vi "launch_auto2_test .vi"(7 "枚举":T1, 8 "error in (no error)":errorcluster, 9 "user event out":T2, 10 "modbusData":refnum<notifier>, 11 "Cluster":T3) -> (0 "error out":errorcluster)   [LabVIEW 2019]
uses:
  core_dataRefCluster.ctl
  core_dataRef.ctl
  core_dataCluster.ctl
  instrument/instr_dataCluster.ctl
  gui/test_result_user_event.ctl
  core_autoMonitorDataCluster.ctl
  gui/Enum.ctl
  instrument/Instrument.lvclass
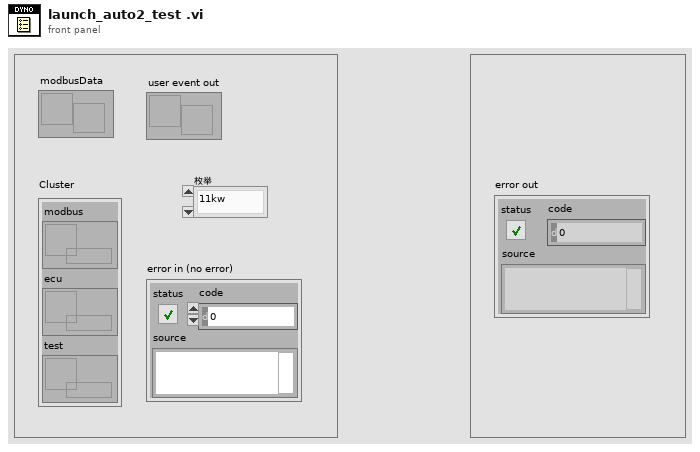
[diagram p1: front panel]
types:
  T1 = typedef "Enum.ctl" = enum16{"11kw", "5KW", "3.5KW"}
  T2 = typedef "test_result_user_event.ctl" = refnum<user-event>
  T3 = typedef "core_dataRefCluster.ctl" = cluster{"modbus":T4, "ecu":T4, "test":T4}
  T4 = typedef "core_dataRef.ctl" = refnum<queue>
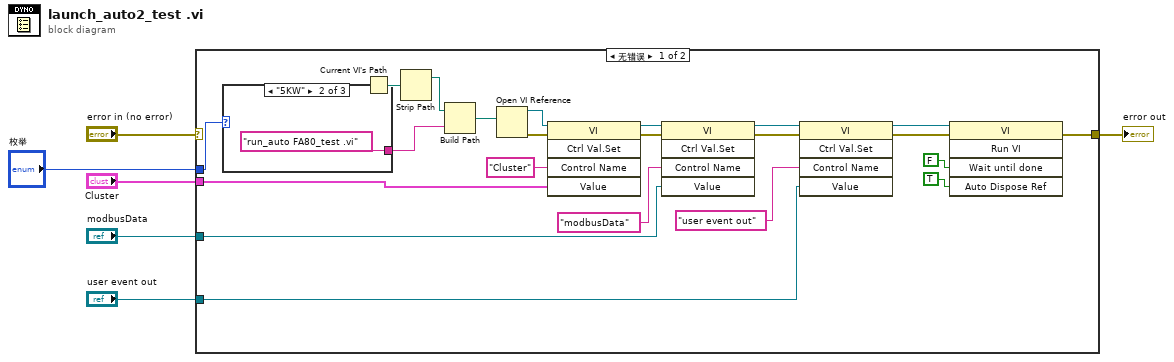
[diagram p0: block diagram]
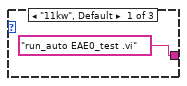
[diagram p2: hidden frame]
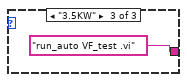
[diagram p3: hidden frame]
diagram:
  n1 = case shown="无错误" "error in (no error)" {
    selector: "error in (no error)" -> [_ w32]
    tunnel: "Cluster" -> [w26 _]
    tunnel: "modbusData" -> [w25 _]
    tunnel: [w15 w32] -> w4
    tunnel: "user event out" -> [w9 _]
    tunnel: "枚举" -> [w7 _]
    frame No Error {
      n2 = case shown="\"5KW\"" w7 {
        tunnel: ["run_auto EAE0_test .vi" ("name or relative path") "run_auto FA80_test .vi" ("name or relative path") "run_auto VF_test .vi" ("name or relative path")] -> w14
        frame "11kw", Default {
        }
        frame "5KW" {
        }
        frame "3.5KW" {
        }
      }
      n3 = Current VI's Path() -> (path=w22:path)
      n4 = Strip Path(path=w22) -> (stripped path=w21:path)  [unwired: 1 out]
      n5 = Build Path(base path=w21, name or relative path=w14) -> (appended path=w20:path)
      n6 = Open VI Reference(vi path=w20) -> (vi reference=w28:refnum<vi>, error out=w23:errorcluster)  [unwired: 5 in]
      n7 = invoke class="VI" method="Ctrl Val.Set"(reference=w28, error in=w23, "Control Name"="Cluster", "Value"=w26) -> (reference out=w27:refnum<vi>, error out=w24:errorcluster)  [unwired: 1 in, 3 out]
      n8 = invoke class="VI" method="Ctrl Val.Set"(reference=w27, error in=w24, "Control Name"="modbusData", "Value"=w25) -> (reference out=w13:refnum<vi>, error out=w11:errorcluster)  [unwired: 1 in, 3 out]
      n9 = invoke class="VI" method="Ctrl Val.Set"(reference=w13, error in=w11, "Control Name"="user event out", "Value"=w9) -> (reference out=w12:refnum<vi>, error out=w10:errorcluster)  [unwired: 1 in, 3 out]
      n10 = invoke class="VI" method="Run VI"(reference=w12, error in=w10, "Wait until done"=FALSE ("Wait Until Done"), "Auto Dispose Ref"=TRUE ("Auto Dispose Reference")) -> (error out=w15:errorcluster)  [unwired: 1 in, 4 out]
    }
    frame Error {
    }
  }
  "error out" <- w4
